vi "Terminate.vi"(8 "error in (no error)":errorcluster, 10 "Message in":refnum<class "TerminateMessage.lvclass">, 11 "focus in":refnum<class "focus.lvclass">) -> (0 "error out":errorcluster, 3 "focus out":refnum<class "focus.lvclass">)   [LabVIEW 2012, in "focus.lvclass"]
doc: "This member function is called when the statemachine in the run.vi receives an 'terminate' command. It closes the RabbitMQ connection. \n\nOverride this member function in your derived class to release all previously acquired resources (but don't forget to call the parent method). If your component has subcomponents, they count as resources, and you have to release them by calling their own terminate functions."
uses:
  focus.lvclass
  <vilib>/Distrio/Murmex/TerminateMessage/TerminateMessage.lvclass
  <vilib>/Distrio/Murmex/Murmex/Murmex.lvclass
panel:
  out "Array":bool[](array[boolean])
  # "This method is called when the TERMINATE\ntrigger is sent. \n\nOverride this method when your component needs to\nrespond to this trigger. \n\nCall parent for proper implementation"
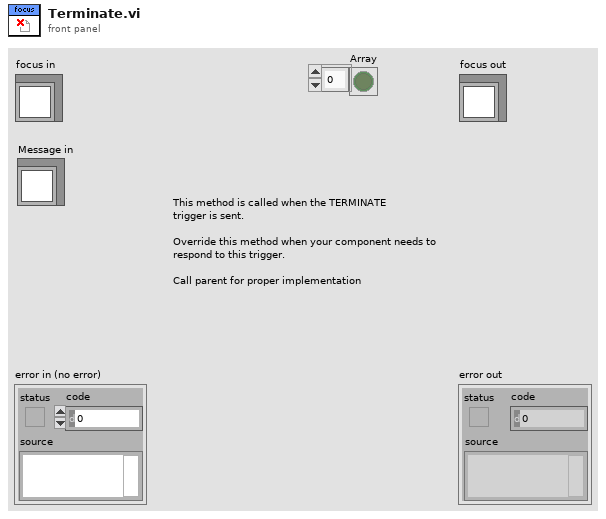
[diagram p1: front panel]
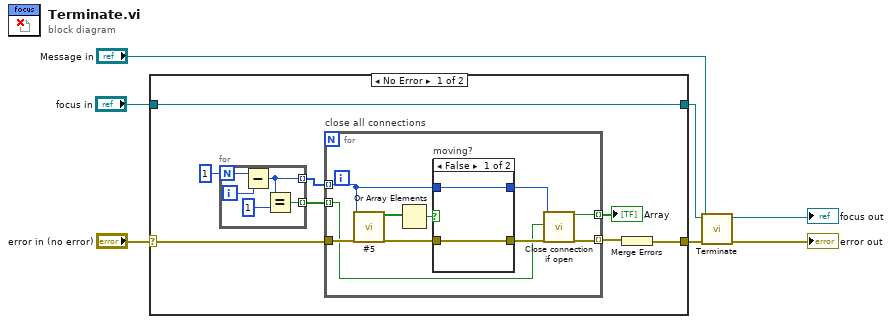
[diagram p0: block diagram]
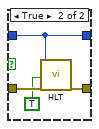
[diagram p2: hidden frame]
diagram:
  n1 = case shown="No Error" "error in (no error)" {
    selector: "error in (no error)" -> [w14 w37]
    tunnel: [w9 w37] -> w4
    tunnel: "focus in" -> [w8 w38]
    tunnel: [w8 w38] -> w2
    frame No Error {
      n2 = for {
        N: 1 -> [w36]
        tunnel: [w34] -> w13 mode=indexing
        tunnel: [w32] -> w12 mode=indexing
        i -> [w35]
        n3 = Subtract(x=w36, y=w35) -> (x-y=w34:i32)
        n4 = Equal?(x=w34, y=1) -> (x = y?=w32:bool)
      }
      n5 = for "close all connections" {
        tunnel: w14 -> [w25]
        tunnel: w13 -> [w21] mode=indexing
        tunnel: w12 -> [w16] mode=indexing
        tunnel: [w18] -> w10 mode=indexing
        tunnel: [w17] -> w11 mode=indexing
        n6 = call "#5.vi"("System no."=w21, "error in"=w25) -> ("Axis moving?"=w24:bool[], "error out"=w22:errorcluster)  [unwired: 16 in]
        n7 = Or Array Elements(Boolean array=w24) -> (logical OR=w23:bool)
        n8 = case "moving?" shown="False" w23 {
          tunnel: w22 -> [w26 w31]
          tunnel: [w26 w30] -> w19
          tunnel: w21 -> [w27 w28]
          tunnel: [w27 w28] -> w20
          frame False {
          }
          frame True {
            n9 = call "HLT.vi"("System no."=w28, "All axes?"=TRUE ("all axes"), "error in"=w31) -> ("error out"=w30:errorcluster)  [unwired: 16 in]
          }
        }
        n10 = call "Close connection if open.vi"("System no."=w20, "Close DaisyChain"=w16, "error in"=w19) -> ("Was connected?"=w17:bool, "error out"=w18:errorcluster)  [unwired: 15 in]
      }
      "Array" <- w11
      n11 = Merge Errors(w10) -> (w9:errorcluster)
    }
    frame Error {
    }
  }
  n12 = call-parent "Terminate.vi"("error in (no error)"=w4, "Message in"="Message in", "Murmex in"=w2) -> ("error out"=→"error out":errorcluster, "Murmex out"=→"focus out":refnum<class "focus.lvclass">)  [unwired: 7 in]
